vi "Confidence Interval (Gauss).vi"(0 "Y":dbl[](array[numeric]), 1 "confidence level":dbl=0.95, 5 "X":dbl[](array[numeric]), 7 "Weight":dbl[](array[numeric]), 9 "amplitude":dbl, 11 "center":dbl, 12 "standard deviation":dbl) -> (4 "Upper Bound":dbl[](array[numeric]), 6 "Lower Bound":dbl[](array[numeric]), 8 "delta amplitude":dbl, 10 "delta center":dbl, 14 "delta standard deviation":dbl, 15 "error":i32)   [LabVIEW 2014, in "NI_AALPro.lvlib"]
doc: "Calculates statistical intervals of the best Gaussian fit for a data set (<B>X</B>, <B>Y</B>). You must manually select the polymorphic instance to use."
uses:
  NI_AALPro.lvlib
  lvanlys.dll
panel:
  out "Coef. Lower Bound":dbl[](array[numeric])
  out "Coef. Upper Bound":dbl[](array[numeric])
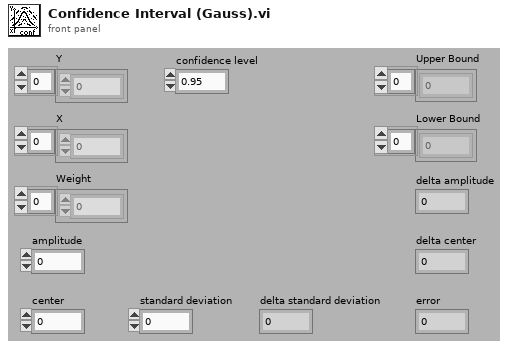
[diagram p1: front panel]
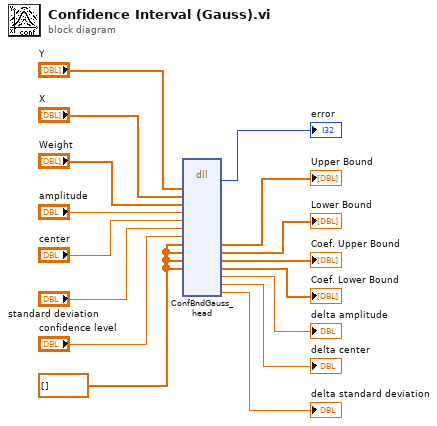
[diagram p0: block diagram]
diagram:
  w10 = dbl[] [] ("Coefficients (Upper)")
  n1 = dll-call lib="C:/Program Files (x86)/National Instruments/LabVIEW 2014/resource/lvanlys.*" fn="ConfBndGauss_head"("y"="Y", "x"="X", "weight"="Weight", "amplitude"="amplitude", "center"="center", "width"="standard deviation", "confidentLevel"="confidence level", "upper"=w10, "lower"=w10, "upperCoef"=w10, "lowerCoef"=w10) -> (→"error":i32, "upper"=→"Upper Bound":dbl[], "lower"=→"Lower Bound":dbl[], "upperCoef"=→"Coef. Upper Bound":dbl[], "lowerCoef"=→"Coef. Lower Bound":dbl[], "deltaAmp"=→"delta amplitude":dbl, "deltaCnt"=→"delta center":dbl, "deltaDev"=→"delta standard deviation":dbl)  [unwired: 13 in, 2 out]
